vi "Measurement Data Convert.vi"   [LabVIEW 2021, in "Yokogawa WT1800 Series.lvlib"]
doc: "Transforms measurement datas into numeric values."
uses:
  <instrlib>/Yokogawa WT1800 Series/Yokogawa WT1800 Series.lvlib
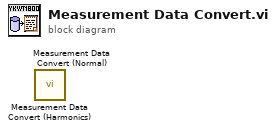
[diagram p0: block diagram]
diagram:
  n1 = call <instrlib>:"Measurement Data Convert (Harmonics).vi"() -> ()  [unwired: 8 in, 4 out]
  n2 = call <instrlib>:"Measurement Data Convert (Normal).vi"() -> ()  [unwired: 8 in, 4 out]
